vi "detectVarables.vi"(3 "error in (no error)":errorcluster, 4 "PortIP":string, 5 "VISA resource name":refnum<visa-resource-name>="COM1" caption="端口号") -> (0 "error out":errorcluster, 1 "Data":string, 2 "VISA resource name 2":refnum<visa-resource-name>="COM1" caption="端口号")   [LabVIEW 2010]
uses:
  GlobalCostants.vi
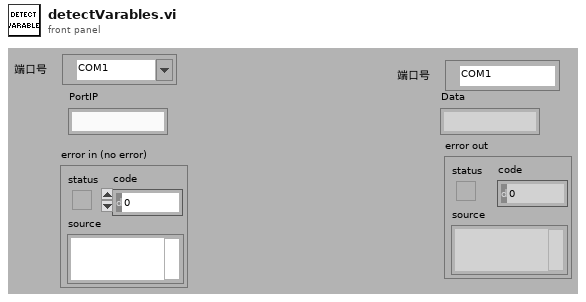
[diagram p1: front panel]
types:
  T1 = typedef "VarableStruct.ctl" = cluster{"Name":string, "StorageRefnum":refnum<file>, "Command":string, "IsDetecting":bool, "VarableID":T2}
  T2 = typedef "VarableID.ctl" = enum16{"current", "voltage", "power", "PF"}
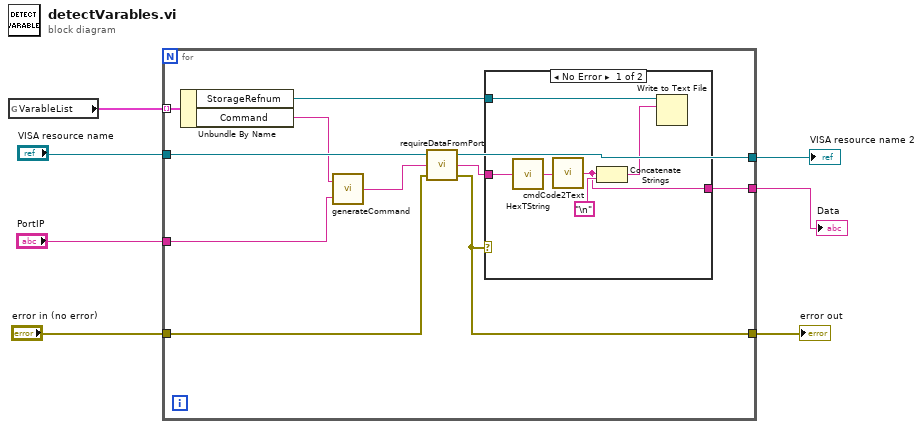
[diagram p0: block diagram]
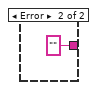
[diagram p2: hidden frame]
diagram:
  n1 = global read "GlobalCostants.vi" "VarableList"() -> (w7:T1[])
  n2 = for {
    tunnel: w7 -> [w15] mode=indexing
    tunnel: "VISA resource name" -> [w18]
    tunnel: [w17] -> w5
    tunnel: "error in (no error)" -> [w13]
    tunnel: [w12] -> w3
    tunnel: "PortIP" -> [w10]
    tunnel: [w8] -> w1
    n3 = Unbundle By Name(w15) -> ("StorageRefnum"=w16:refnum<file>, "Command"=w11:string)
    n4 = call "generateCommand.vi"("IP"=w10, "CommandProtoType"=w11) -> ("Command"=w9:string)
    n5 = call "requireDataFromPort.vi"("error in (no error)"=w13, "Command"=w9, "VISA resource name"=w18) -> ("error out"=w12:errorcluster, "Data"=w14:string, "VISA resource name 2"=w17:refnum<visa-resource-name>)
    n6 = case shown="No Error" w12 {
      tunnel: w16 -> [w24 _]
      tunnel: w14 -> [w22 _]
      tunnel: [w19 "" ("数据字符串")] -> w8
      frame No Error {
        n7 = call "HexTString.vi"("input Hex"=w22) -> ("output string"=w20:string)
        n8 = call "cmdCode2Text.vi"("CommandCode"=w20) -> ("CommandText"=w19:string)
        n9 = Concatenate Strings(w19, "\n") -> (w21:string)
        n10 = Write to Text File(file (use dialog)=w24, text=w21) -> ()  [unwired: 2 in, 3 out]
      }
      frame Error {
      }
    }
  }
  "VISA resource name 2" <- w5
  "error out" <- w3
  "Data" <- w1
